vi "epx_Update Display State.vi"(10 "Display State In":T2={"BGColor"=0, "FGColor"=0, "GridColor"=9868950, "Number of Polar Grids"=12, "Number of Circle Grids"=4, "Vector.Active"=0, "Vectors.Properties"=[], "Height"=0, "Width"=0} {"Number of Circle Grids" min=1 max=100 step=1; "Number of Polar Grids" min=1 max=100 step=1}, 11 "Data In":T1) -> (1 "State Changed?":bool, 2 "Display State Out":T2={"BGColor"=0, "FGColor"=0, "GridColor"=9868950, "Number of Polar Grids"=12, "Number of Circle Grids"=4, "Vector.Active"=0, "Vectors.Properties"=[], "Height"=0, "Width"=0} {"Number of Circle Grids" min=1 max=100 step=1; "Number of Polar Grids" min=1 max=100 step=1})   [LabVIEW 2011, in "NI_EP_Basic.lvlib" / "EPX Vector Diagram.xctl"]
uses:
  <vilib>/addons/Electrical Power/Basic/Controls/Vector Diagram/EPX Vector Diagram.xctl
  <vilib>/addons/Electrical Power/Basic/Controls/Vector Diagram/Abilities/epx_Vector Diagram State.ctl
  <vilib>/addons/Electrical Power/Basic/Controls/Vector Diagram/SubVIs/epx_Vector Type.ctl
  <vilib>/addons/Electrical Power/Basic/Controls/Vector Diagram/Abilities/epx_Vector Diagram Data.ctl
  <vilib>/addons/Electrical Power/Basic/NI_EP_Basic.lvlib
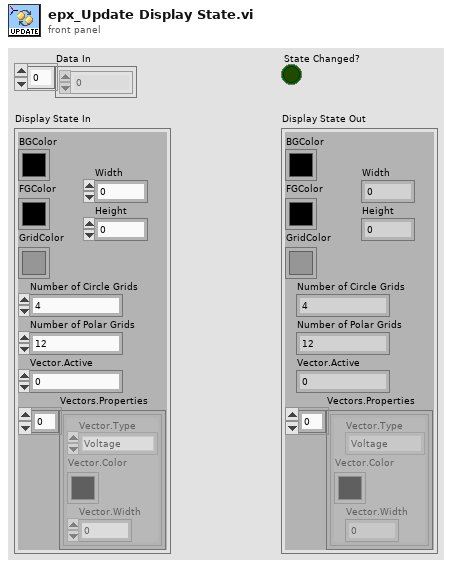
[diagram p1: front panel]
types:
  T1 = typedef "NI_EP_Basic.lvlib/EPX Vector Diagram.xctl/epx_Vector Diagram Data.ctl" = cdb[]
  T2 = typedef "NI_EP_Basic.lvlib/EPX Vector Diagram.xctl/epx_Vector Diagram State.ctl" = cluster{"BGColor":u32, "FGColor":u32, "GridColor":u32, "Number of Polar Grids":i32, "Number of Circle Grids":i32, "Vector.Active":i32, "Vectors.Properties":cluster{"Vector.Type":T3, "Vector.Color":u32, "Vector.Width":u8}[], "Height":u32, "Width":u32}
  T3 = typedef "NI_EP_Basic.lvlib/epx_Vector Type.ctl" = enum16{"Voltage", "Current"}
  T4 = cluster{"Vector.Type":T3, "Vector.Color":u32, "Vector.Width":u8}[]
  T5 = cluster{"Vector.Type":T3, "Vector.Color":u32, "Vector.Width":u8}
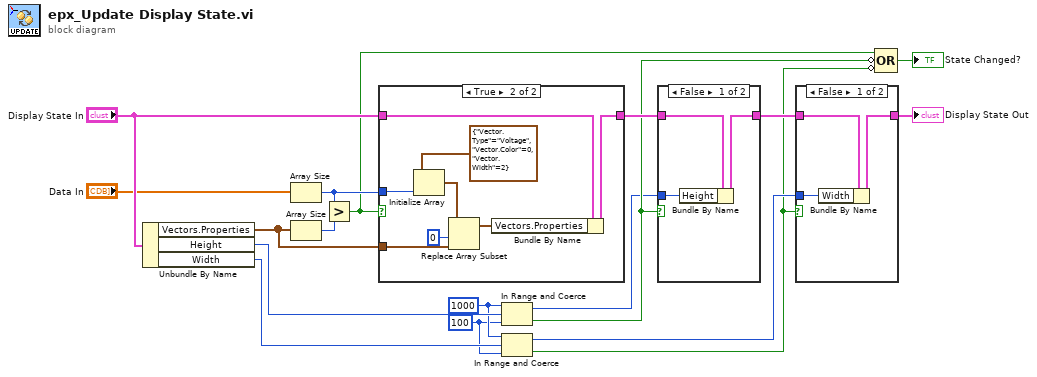
[diagram p0: block diagram]
diagram:
  w10 = u32 100 ("lower limit")
  w11 = u32 1000 ("upper limit")
  n1 = Unbundle By Name("Display State In") -> ("Vectors.Properties"=w16:T4, "Height"=w13:u32, "Width"=w12:u32)
  n2 = Array Size(array="Data In") -> (size(s)=w17:i32)
  n3 = Array Size(array=w16) -> (size(s)=w18:i32)
  n4 = Greater?(x=w17, y=w18) -> (0:w9:bool)
  n5 = case shown="True" w9 {
    tunnel: [w19 w22] -> w7
    tunnel: "Display State In" -> [w19 w23]
    tunnel: w17 -> [_ w27]
    tunnel: w16 -> [_ w25]
    frame False {
    }
    frame True {
      n6 = Initialize Array(T5 {"Vector.Type"=enum."Voltage", "Vector.Color"=0, "Vector.Width"=2} ("Vector.Properties"), w27) -> (w26:T4)
      n7 = Replace Array Subset(array=w26, new element=w25, index=0) -> (w21:T4)
      n8 = Bundle By Name(cluster=w23, "Vectors.Properties"=w21) -> (w22:T2)
    }
  }
  n9 = In Range and Coerce(upper limit=w11, x=w13, lower limit=w10) -> (coerced(x)=w5:u32, In Range?=w6:bool)
  n10 = In Range and Coerce(upper limit=w11, x=w12, lower limit=w10) -> (coerced(x)=w2:u32, In Range?=w1:bool)
  n11 = case shown="False" w6 {
    tunnel: [w29 w31] -> w4
    tunnel: w7 -> [w30 w31]
    tunnel: w5 -> [w28 _]
    frame False {
      n12 = Bundle By Name(cluster=w30, "Height"=w28) -> (w29:T2)
    }
    frame True {
    }
  }
  n13 = case shown="False" w1 {
    tunnel: [w33 w35] -> w3
    tunnel: w4 -> [w34 w35]
    tunnel: w2 -> [w32 _]
    frame False {
      n14 = Bundle By Name(cluster=w34, "Width"=w32) -> (w33:T2)
    }
    frame True {
    }
  }
  "Display State Out" <- w3
  n15 = Compound Arithmetic op=OR(w9, invert w6, invert w1) -> (→"State Changed?":bool)
